vi "camera button switching.vi"(8 "Cam 2 Button":bool, 11 "Cam 1 Button":bool) -> (3 "Use Cam 2?":bool)   [LabVIEW 2015]
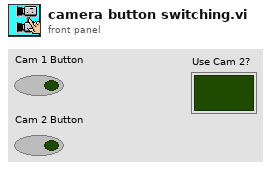
[diagram p1: front panel]
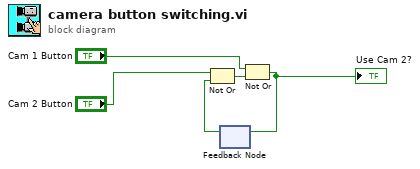
[diagram p0: block diagram]
diagram:
  n1 = feedback #1() -> (w2:bool)  [unwired: 1 in]
  n2 = Not Or(1:w2, 2:"Cam 2 Button") -> (0:w5:bool)
  n3 = Not Or(1:w5, 2:"Cam 1 Button") -> (0:w1:bool)
  "Use Cam 2?" <- w1
  n4 = feedback-in #1(w1) -> ()
